vi "LoadDeviceImage.vi"(11 "DevID":u32) -> (2 "AppBGpic":picture, 3 "Image Found?":bool=TRUE)   [LabVIEW 2015]
uses:
  <vilib>/picture/picture.llb/Draw True-Color Pixmap.vi
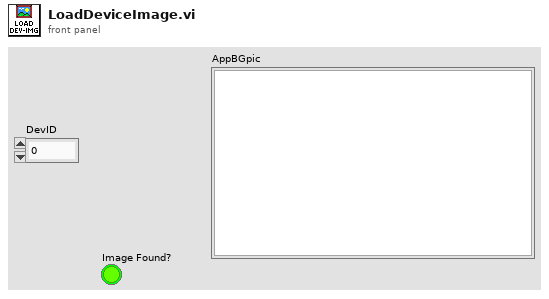
[diagram p1: front panel]
types:
  T1 = typedef "imagedata.ctl" = cluster{"image type":i32, "image depth":i32, "image":u8[], "mask":u8[], "colors":u32[], "Rectangle":cluster{"left":i16, "top":i16, "right":i16, "bottom":i16}}
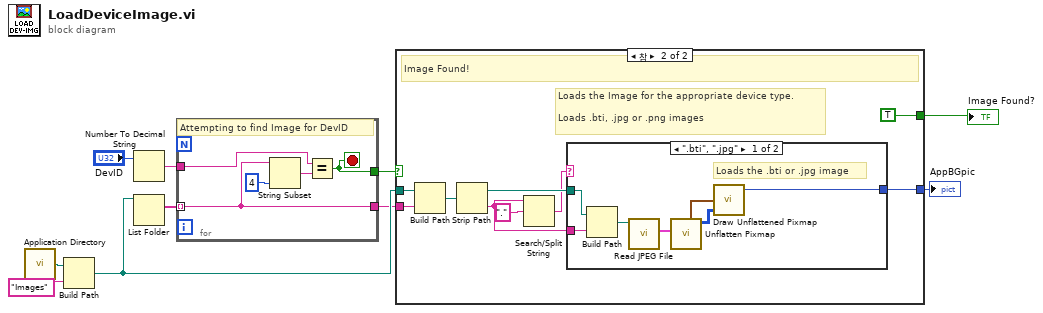
[diagram p0: block diagram]
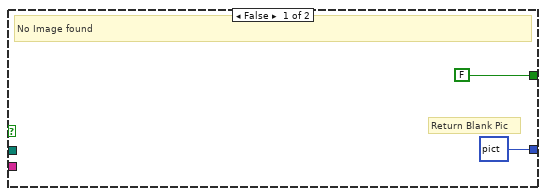
[diagram p2: hidden frame]
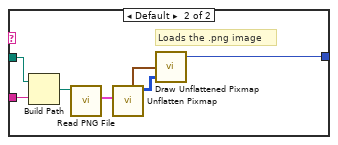
[diagram p3: hidden frame]
diagram:
  n1 = call <vilib>:"Application Directory.vi"() -> ("Application Directory"=w10:path)
  n2 = Build Path(base path=w10, name or relative path="Images") -> (appended path=w4:path)
  n3 = Number To Decimal String(number="DevID") -> (decimal integer string=w6:string)  [unwired: 1 in]
  n4 = List Folder(path=w4) -> (filenames=w7:string[])  [unwired: 3 in, 3 out]
  n5 = for {
    tunnel: w7 -> [w12] mode=indexing
    tunnel: w6 -> [w14]
    tunnel: [w12] -> w3
    tunnel: [w11] -> w2
    stop <- w11 stop-if-true
    # "Attempting to find Image for DevID"
    n6 = String Subset(string=w12, length (rest)=4 ("length (rest)")) -> (substring=w13:string)  [unwired: 1 in]
    n7 = Equal?(x=w14, y=w13) -> (x = y?=w11:bool)
  }
  n8 = case shown="참" w2 {
    tunnel: [picture data[5B] ("new picture") w26] -> w5
    tunnel: w4 -> [_ w25]
    tunnel: w3 -> [_ w24]
    tunnel: [FALSE ("Boolean") TRUE ("Boolean")] -> w1
    frame False {
      # "Return Blank Pic"
      # "No Image found"
    }
    frame True {
      # "Loads the Image for the appropriate device type. \n\nLoads .bti, .jpg or .png images"
      # "Image Found!"
      n9 = Build Path(base path=w25, name or relative path=w24) -> (appended path=w19:path)
      n10 = Strip Path(path=w19) -> (stripped path=w23:path, name=w22:string)
      n11 = Search/Split String(string=w22, search string/char (-)=".") -> (match + rest of string=w20:string)  [unwired: 1 in, 2 out]
      n12 = case shown="\".bti\", \".jpg\"" w20 {
        tunnel: w23 -> [w30 w38]
        tunnel: [w32 w40] -> w26
        tunnel: w22 -> [w31 w37]
        frame ".bti", ".jpg" {
          # "Loads the .bti or .jpg image"
          n13 = Build Path(base path=w30, name or relative path=w31) -> (appended path=w33:path)
          n14 = call <vilib>:"Read JPEG File.vi"("path to JPEG file"=w33) -> ("image data"=w29:T1)  [unwired: 8 in, 2 out]
          n15 = call <vilib>:"Unflatten Pixmap.vi"("image data"=w29) -> ("24-bit pixmap"=w27:u32[][], "top left"=w28:cluster{"x":i16, "y":i16})  [unwired: 4 in, 5 out]
          n16 = call-poly <vilib>:"Draw Unflattened Pixmap.vi"("top left point(0, 0)"=w28, "data (RGB format)"=w27) -> ("new picture"=w32:picture)  [unwired: 7 in]
        }
        frame Default {
          # "Loads the .png image"
          n17 = Build Path(base path=w38, name or relative path=w37) -> (appended path=w39:path)
          n18 = call <vilib>:"Read PNG File.vi"("path to PNG file"=w39) -> ("image data"=w34:T1)  [unwired: 8 in, 2 out]
          n19 = call <vilib>:"Unflatten Pixmap.vi"("image data"=w34) -> ("24-bit pixmap"=w35:u32[][], "top left"=w36:cluster{"x":i16, "y":i16})  [unwired: 4 in, 5 out]
          n20 = call-poly <vilib>:"Draw Unflattened Pixmap.vi"("top left point(0, 0)"=w36, "data (RGB format)"=w35) -> ("new picture"=w40:picture)  [unwired: 7 in]
        }
      }
    }
  }
  "AppBGpic" <- w5
  "Image Found?" <- w1
